vi "TransferFunction.vi"(7 "Limit Cluster":cluster{"Upper Limit":dbl, "Lower Limit":dbl}, 8 "error in (no error)":errorcluster, 10 "Sampling Time (s)":dbl format="%#.6p", 11 "Cluster":T2) -> (0 "error out":errorcluster, 2 "Transfer Function":T1={"Transfer Function"={"Numerator"=[1.0], "Denominator"=[-0.9, 1.0]}, "Limit Cluster"={"Upper Limit"=0.0, "Lower Limit"=0.0}}, 3 "Transfer Function Model":T3 {"transfer function(s)"."delay" format="%.4f"; "transfer function(s)"."Denominator" format="%#_3g"; "transfer function(s)"."Numerator" format="%#_3g"; "properties"."Sampling Time" format="%#.6p"; "properties"."Output Delays" format="%.4f"; "properties"."Input Delays" format="%.4f"})   [LabVIEW 2020]
uses:
  <vilib>/addons/Control Design/_Model Construction/Model Typedefs.llb/CD Transfer Function Model (MIMO).ctl
  <vilib>/addons/Control Design/_Model Construction/Model Typedefs.llb/CD General Elements.ctl
  <vilib>/addons/Control Design/_Model Construction/Model Typedefs.llb/CD Transfer Function Model (SISO).ctl
  Controls/TFspec.ctl
  Controls/controlspec.ctl
  <vilib>/addons/Control Design/_Model Construction/Model Creation.llb/Model Creation SubVI/cd_Create Transfer Function Model.vi
  <vilib>/addons/Control Design/_Model Construction/Model Information.llb/Model Information SubVIs/cd_Get Num Den From TF Model.vi
  <vilib>/addons/Control Design/_Model Construction/NI_LinSys_Model Creation.lvlib
  <vilib>/addons/Control Design/_Model Construction/NI_LinSys_Model Information.lvlib
  <vilib>/addons/Control Design/_Model Construction/NI_LinSys_Model Typedefs.lvlib
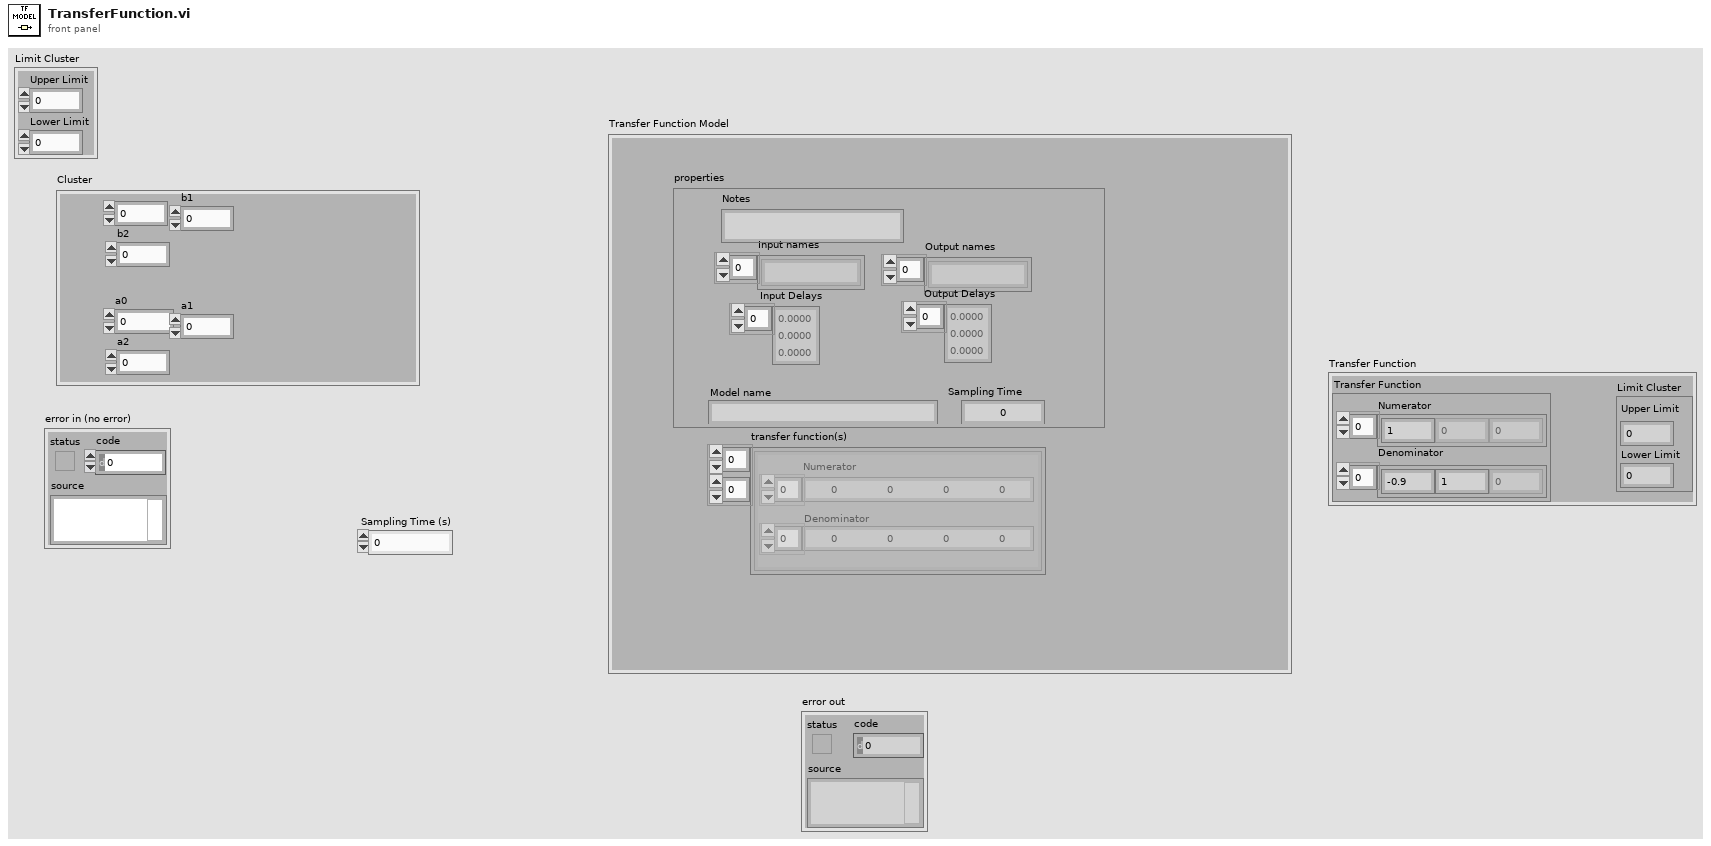
[diagram p1: front panel]
types:
  T1 = typedef "controlspec.ctl" = cluster{"Transfer Function":cluster{"Numerator":dbl[], "Denominator":dbl[]}, "Limit Cluster":cluster{"Upper Limit":dbl, "Lower Limit":dbl}}
  T2 = typedef "TFspec.ctl" = cluster{"b0":dbl, "b1":dbl, "b2":dbl, "a0":dbl, "a1":dbl, "a2":dbl}
  T3 = typedef "NI_LinSys_Model Typedefs.lvlib/CD Transfer Function Model (MIMO).ctl" = cluster{"properties":T4, "transfer function(s)":T5[][]}
  T4 = typedef "NI_LinSys_Model Typedefs.lvlib/CD General Elements.ctl" = cluster{"Model name":string, "Input names":string[], "Output names":string[], "Input Delays":dbl[], "Output Delays":dbl[], "Sampling Time":dbl, "Notes":string}
  T5 = typedef "NI_LinSys_Model Typedefs.lvlib/CD Transfer Function Model (SISO).ctl" = cluster{"Numerator":dbl[], "Denominator":dbl[], "delay":dbl}
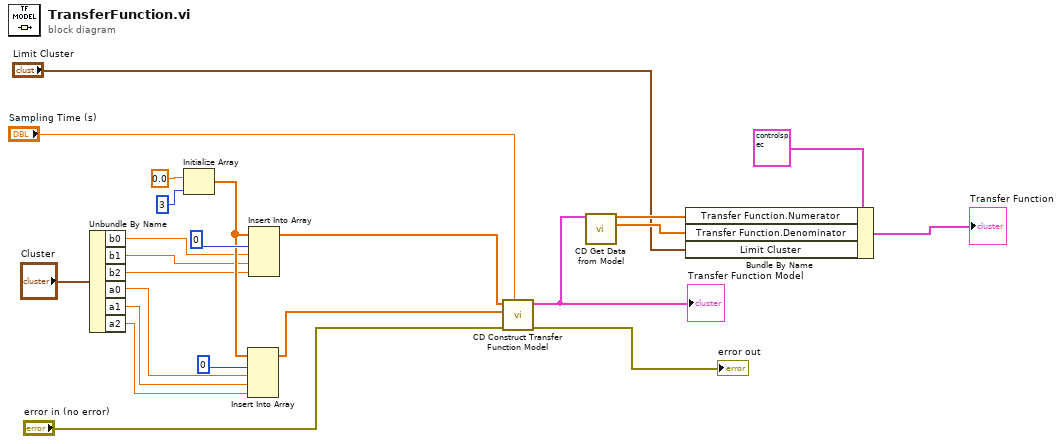
[diagram p0: block diagram]
diagram:
  n1 = Unbundle By Name("Cluster") -> ("b0"=w16:dbl, "b1"=w15:dbl, "b2"=w14:dbl, "a0"=w13:dbl, "a1"=w12:dbl, "a2"=w11:dbl)
  n2 = Initialize Array(0.0 ("element"), 3 ("dimension size")) -> (w19:dbl[])
  n3 = Insert Into Array(array=w19, index=0, new element #1=w13, new element #2=w12, new element #3=w11) -> (w18:dbl[])
  n4 = Insert Into Array(array=w19, index=0, new element #1=w16, new element #2=w15, new element #3=w14) -> (w20:dbl[])
  n5 = call-poly <vilib>:"CD Construct Transfer Function Model.vi"("Sampling Time (s)"="Sampling Time (s)", "error in (no error)"="error in (no error)", "Denominator"=w18, "Numerator"=w20) -> ("error out"=→"error out":errorcluster, "Transfer Function Model"=w6:T3)  [unwired: 6 in]
  "Transfer Function Model" <- w6
  n6 = call-poly <vilib>:"CD Get Data from Model.vi"("Transfer Function Model"=w6) -> ("Numerator"=w4:dbl[], "Denominator"=w3:dbl[])  [unwired: 11 in, 2 out]
  n7 = Bundle By Name(cluster=T1 {"Transfer Function"={"Numerator"=[1.0], "Denominator"=[-0.9, 1.0]}, "Limit Cluster"={"Upper Limit"=0.0, "Lower Limit"=0.0}}, "Transfer Function.Numerator"=w4, "Transfer Function.Denominator"=w3, "Limit Cluster"="Limit Cluster") -> (→"Transfer Function":T1)
